vi "Begin.vi"(11 "Image Size":T1=enum."160x120") -> (0 "error out":errorcluster)   [LabVIEW 2011]
doc: "Called before other user functions, this VI is expected to open initial I/O refnums, load in file data, and do all program initialization. Notice that the <B>error out</B> terminal is simply used for data flow. Wiring it to other structures or subVIs ensures that this VI runs first."
uses:
  <vilib>/Rock Robotics/WPI/Camera/WPI_CameraImageSize.ctl
  <vilib>/Rock Robotics/SystemInterfaces/DIO/FPGA_DIOPWMChannel.ctl
  <vilib>/Rock Robotics/WPI/Joystick/WPI_JoystickDeviceEnum.ctl
  <vilib>/Rock Robotics/WPI/Camera/WPI_CameraWhite Balance Values.ctl
  <vilib>/Rock Robotics/WPI/Camera/WPI_CameraExposure Values.ctl
  <vilib>/Rock Robotics/WPI/Camera/WPI_CameraFrameRate.ctl
  <vilib>/Rock Robotics/SystemInterfaces/DIO/FPGA_DIOChannel.ctl
  <vilib>/Rock Robotics/SystemInterfaces/Typedef/FPGA_TypedefDigitalModule.ctl
  <vilib>/Rock Robotics/WPI/Encoder/WPI_EncoderType.ctl
  <vilib>/Rock Robotics/SystemInterfaces/DIO/FPGA_DIORelayChannel.ctl
  <vilib>/Rock Robotics/SystemInterfaces/Typedef/FPGA_TypedefAnalogModuleForGyro.ctl
  <vilib>/Rock Robotics/SystemInterfaces/AI/FPGA_AIGyroChannel.ctl
  <vilib>/Rock Robotics/WPI/Relay/WPI_RelayDirection.ctl
  <vilib>/Rock Robotics/WPI/MotorControl/WPI_MotorControlOpen Victor.vi
  <vilib>/Rock Robotics/WPI/RobotDrive/WPI_RobotDriveOpen4MotorWithJaguar.vi
  Robot Global Data.vi
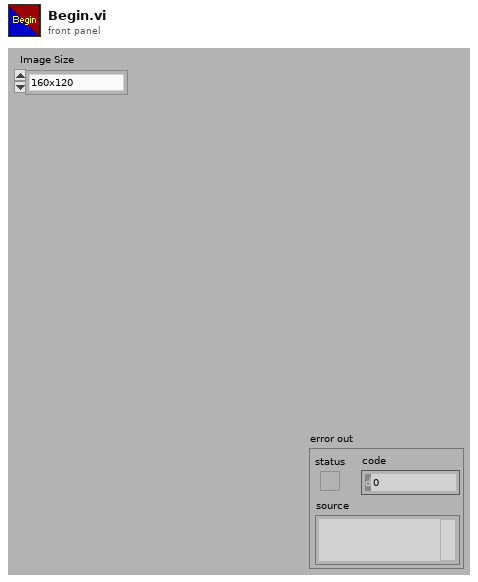
[diagram p1: front panel]
types:
  T1 = typedef "WPI_CameraImageSize.ctl" = enum16{"640x480", "320x240", "160x120"}
  T2 = typedef "WPI_RelayDirection.ctl" = enum16{"Both directions", "Forward only", "Reverse only"}
  T3 = typedef "FPGA_TypedefDigitalModule.ctl" = enum16{"Digital Module 1", "Digital Module 2"}
  T4 = typedef "FPGA_AIGyroChannel.ctl" = enum8{"AI 1", "AI 2", "Invalid"}
  T5 = typedef "FPGA_TypedefAnalogModuleForGyro.ctl" = enum16{"Analog Module 1"}
  T6 = typedef "FPGA_DIORelayChannel.ctl" = enum8{"Relay 1", "Relay 2", "Relay 3", "Relay 4", "Relay 5", "Relay 6", "Relay 7", "Relay 8", "Invalid"}
  T7 = typedef "FPGA_DIOChannel.ctl" = enum8{"DIO 1", "DIO 2", "DIO 3", "DIO 4", "DIO 5", "DIO 6", "DIO 7", "DIO 8", "DIO 9", "DIO 10", "DIO 11", "DIO 12", "DIO 13", "DIO 14", "Invalid"}
  T8 = typedef "WPI_EncoderType.ctl" = enum16{"1x", "2x", "4x"}
  T9 = typedef "FPGA_DIOPWMChannel.ctl" = enum8{"PWM 1", "PWM 2", "PWM 3", "PWM 4", "PWM 5", "PWM 6", "PWM 7", "PWM 8", "PWM 9", "PWM 10", "Invalid"}
  T10 = typedef "WPI_JoystickDeviceEnum.ctl" = enum16{"USB 1", "USB 2", "USB 3", "USB 4", "Kinect 1", "Kinect 2"}
  T11 = typedef "WPI_CameraFrameRate.ctl" = u32
  T12 = typedef "WPI_CameraExposure Values.ctl" = enum16{"Auto", "Flicker-free 50 Hz", "Flicker-free 60 Hz", "Hold current"}
  T13 = typedef "WPI_CameraWhite Balance Values.ctl" = enum16{"Auto", "Fixed indoor", "Fixed outdoor 1", "Fixed outdoor 2", "Fixed fluorescent 1", "Fixed fluorescent 2", "Hold current"}
  T14 = typedef "WPI_CameraDevRef.ctl" = cluster{"Camera Address":string, "CameraStatus":errorcluster, "Acquire Image Notifier":refnum<notifier>}
  T15 = typedef "WPI_DigitalInputDevRef.ctl" = cluster{"DevStatus":errorcluster, "DIO Channel":T7, "Digital Module":T3}
  T16 = typedef "FPGA_CounterEncoderSourceConvertionLVSourceType.ctl" = cluster{"DevStatus":errorcluster, "AnalogTriggerMode?":bool, "DigitalMode":cluster{"Digital Module":T3, "DIO Channel":T17}, "AnalogTriggerMode":cluster{"AnalogTriggerIndex":T18, "OutputType":T19}}
  T17 = typedef "FPGA_DIODigitalSourceChannel.ctl" = enum8{"DIO 1", "DIO 2", "DIO 3", "DIO 4", "DIO 5", "DIO 6", "DIO 7", "DIO 8", "DIO 9", "DIO 10", "DIO 11", "DIO 12", "DIO 13", "DIO 14", "Disabled"}
  T18 = typedef "FPGA_AnalogTriggerIndex.ctl" = enum8{"Trig 0", "Trig 1", "Trig 2", "Trig 3", "Trig 4", "Trig 5", "Trig 6", "Trig 7", "Invalid"}
  T19 = typedef "FPGA_AnalogTriggerOutType.ctl" = enum16{"InWindow", "TriggerState", "Rising", "Falling"}
  T20 = typedef "WPI_GyroDevRef.ctl" = cluster{"DevStatus":errorcluster, "Analog Module":T21, "Analog Channel":T22, "Offset":dbl, "Gain (VoltsPerDegree/Second)":dbl}
  T21 = typedef "FPGA_TypedefAnalogModule.ctl" = enum16{"Analog Module 1", "Analog Module 2"}
  T22 = typedef "FPGA_AIChannel.ctl" = enum8{"AI 1", "AI 2", "AI 3", "AI 4", "AI 5", "AI 6", "AI 7", "AI 8", "Invalid"}
  T23 = typedef "WPI_EncoderDevRef.ctl" = cluster{"DevStatus":errorcluster, "EncoderIndex":T24, "CounterIndex":T25, "DistancePerCount":dbl, "Decoding Type":T8}
  T24 = typedef "FPGA_EncoderIdx.ctl" = enum8{"Enc 0", "Enc 1", "Enc 2", "Enc 3", "Invalid"}
  T25 = typedef "FPGA_CounterCtrSystemIndex.ctl" = enum8{"Ctr 0", "Ctr 1", "Ctr 2", "Ctr 3", "Ctr 4", "Ctr 5", "Ctr 6", "Ctr 7", "Invalid"}
  T26 = typedef "WPI_RobotDriveDevRef.ctl" = cluster{"DevStatus":errorcluster, "Motors[]":T27[], "Square Inputs":bool, "Max Output":dbl, "Isochronous":bool}
  T27 = typedef "WPI_MotorControlDeviceRef.ctl" = cluster{"DeviceStatus":errorcluster, "Type":enum16{"PWM", "CAN"}, "PWM":cluster{"Digital Module":T3, "PWM Channel":T9, "DeadBand":T28}, "CAN":cluster{"Device Number":u8, "Control Mode":T29, "Semaphore":T30, "Max Vout":dbl}, "Invert":bool, "TransformRef":T31, "InvTransformRef":T31}
  T28 = typedef "WPI_PWMDeadband.ctl" = cluster{"Name":string, "maxPositivePwm":i32, "minPositivePwm":i32, "centerPwm":i32, "maxNegativePwm":i32, "minNegativePwm":i32, "angularRange":u16}
  T29 = typedef "WPI_CANJaguar_ControlMode.ctl" = enum8{"Percent VBus", "Current", "Speed", "Position", "Voltage"}
  T30 = typedef "Semaphore RefNum" = refnum<k1>
  T31 = typedef "WPI_PWMTransform_ConPane.ctl" = refnum<vi>
  T32 = typedef "WPI_RelayDevRef.ctl" = cluster{"DevStatus":errorcluster, "Relay Channel":T6, "Digital Module":T3, "Relay Direction":T2}
  T33 = typedef "WPI_JoystickDevRef.ctl" = cluster{"Device":T10}
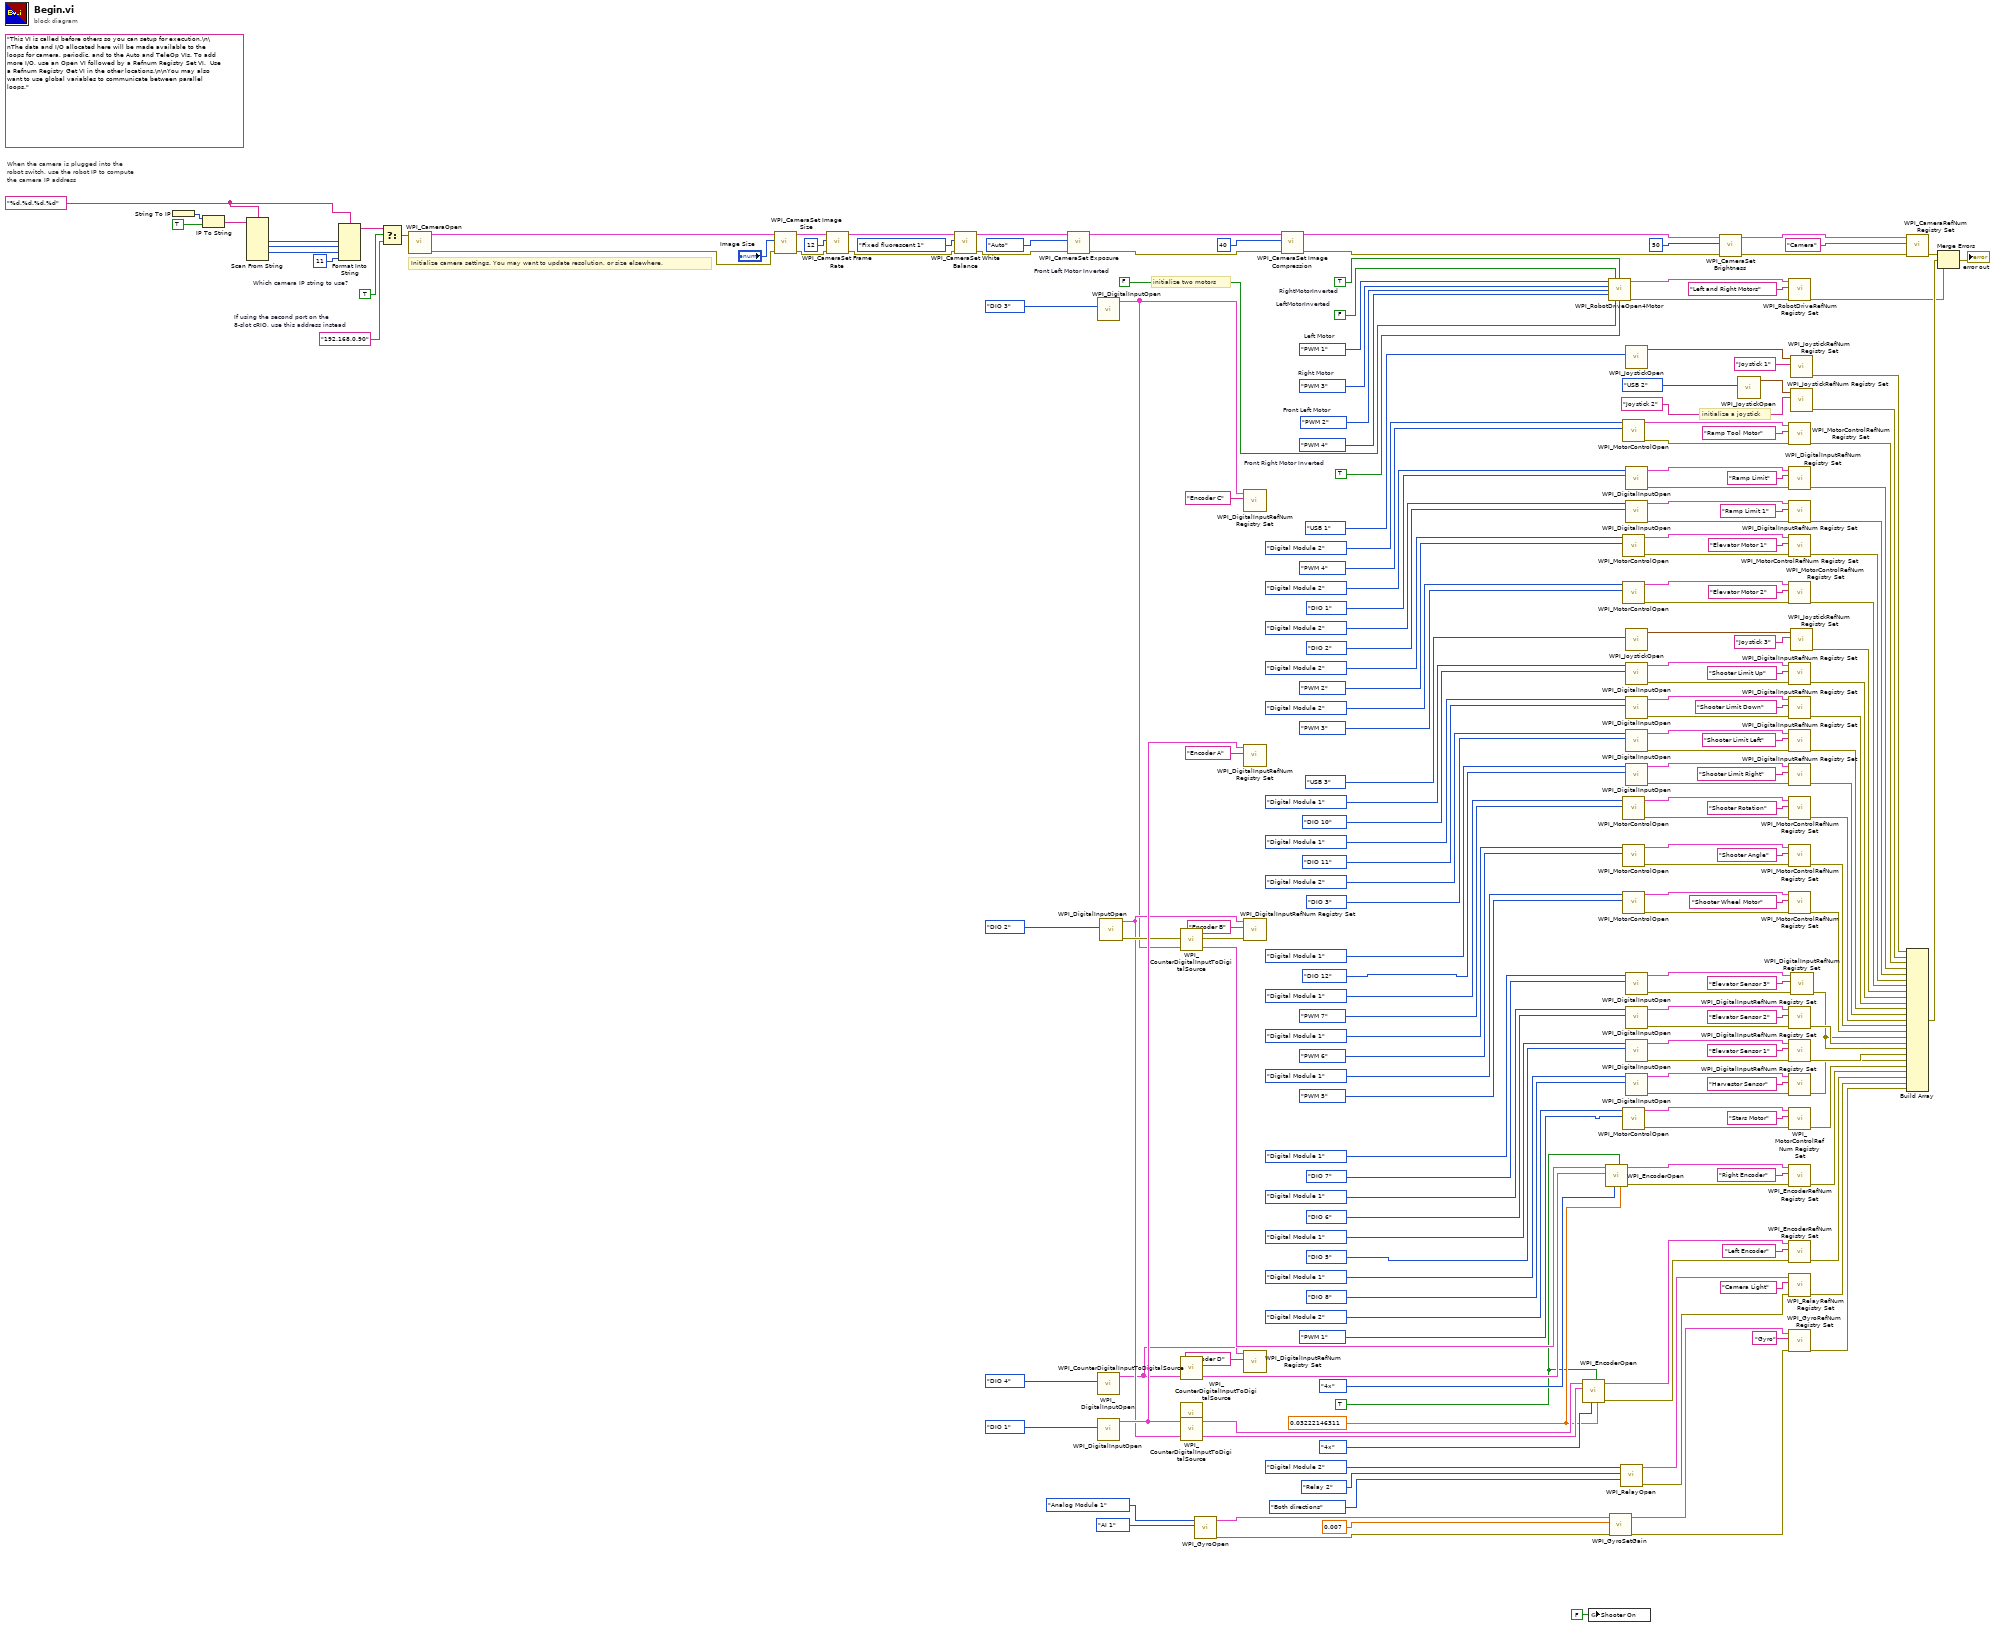
[diagram p0: block diagram]
diagram:
  w10 = FALSE  # Front Left Motor Inverted
  w11 = TRUE  # Front Right Motor Inverted
  w52 = TRUE ("External Reset Active High")
  w62 = 0.03222146311 ("DistancePerCount")
  w148 = FPGA_DIOPWMChannel."PWM 2"  # Front Left Motor
  w166 = TRUE  # Which camera IP string to use?
  w170 = "%d.%d.%d.%d" ("format string")
  (unwired) "This VI is called before others so you can setup for execution.\n\nThe data and I/O allocated here will be made available to the loops for camera, periodic, and to the Auto and TeleOp VIs. To add more I/O, use an Open VI followed by a Refnum Registry Set VI.  Use a Refnum Registry Get VI in the other locations.\n\nYou may also want to use global variables to communicate between parallel loops."
  w182 = FPGA_DIOPWMChannel."PWM 3"  # Right Motor
  w183 = FPGA_DIOPWMChannel."PWM 1"  # Left Motor
  w167 = "192.168.0.90"  # If using the second port on the 8-slot cRIO, use this address instead
  w207 = FALSE  # LeftMotorInverted
  w208 = TRUE  # RightMotorInverted
  # "When the camera is plugged into the\nrobot switch, use the robot IP to compute\nthe camera IP address"
  # "initialize a joystick"
  # "initialize two motors"
  # "Initialize camera settings. You may want to update resolution, or size elsewhere."
  n1 = String To IP() -> (0:w177:u32)  [unwired: 1 in]
  n2 = IP To String(1:TRUE ("dot notation? (F)"), 2:w177) -> (0:w175:string)
  n3 = Scan From String(format string=w170, input string=w175) -> (output 1=w174:i32, output 2=w173:i32, output 3=w172:i32)  [unwired: 7 in, 3 out]
  n4 = Format Into String(format string=w170, w174, w173, w172, 11 ("Compression")) -> (resulting string=w168:string)  [unwired: 2 in, 1 out]
  n5 = Select(t=w168, s=w166, f=w167) -> (s? t:f=w169:string)
  n6 = call <vilib>:"WPI_CameraOpen.vi"("Camera Address"=w169) -> ("error out"=w192:errorcluster, "CameraDevRef"=w193:T14)  [unwired: 1 in, 8 out]
  n7 = call <vilib>:"WPI_CameraSet Image Size.vi"("error in (no error)"=w192, "Image Size"="Image Size", "CameraDevRef"=w193) -> ("error out"=w191:errorcluster, "CameraDevRef Out"=w194:T14)  [unwired: 7 out]
  n8 = call <vilib>:"WPI_CameraSet Frame Rate.vi"("error in (no error)"=w191, "Frame Rate (fps)"=T11 12, "CameraDevRef"=w194) -> ("error out"=w190:errorcluster, "CameraDevRef Out"=w196:T14)  [unwired: 7 out]
  n9 = call <vilib>:"WPI_CameraSet White Balance.vi"("error in (no error)"=w190, "White Balance"=WPI_CameraWhite_Balance_Values."Fixed fluorescent 1", "CameraDevRef"=w196) -> ("error out"=w189:errorcluster, "CameraDevRef Out"=w195:T14)  [unwired: 7 out]
  n10 = call <vilib>:"WPI_CameraSet Exposure.vi"("error in (no error)"=w189, "Exposure"=WPI_CameraExposure_Values."Auto", "CameraDevRef"=w195) -> ("error out"=w188:errorcluster, "CameraDevRef Out"=w198:T14)  [unwired: 7 out]
  n11 = call <vilib>:"WPI_DigitalInputOpen.vi"("DIO Channel"=FPGA_DIOChannel."DIO 3") -> ("DigitalInputDevRef"=w56:T15)  [unwired: 2 in, 8 out]
  n12 = call <vilib>:"WPI_DigitalInputOpen.vi"("DIO Channel"=FPGA_DIOChannel."DIO 4") -> ("DigitalInputDevRef"=w55:T15)  [unwired: 2 in, 8 out]
  n13 = call <vilib>:"WPI_DigitalInputOpen.vi"("DIO Channel"=FPGA_DIOChannel."DIO 1") -> ("DigitalInputDevRef"=w61:T15)  [unwired: 2 in, 8 out]
  n14 = call <vilib>:"WPI_DigitalInputOpen.vi"("DIO Channel"=FPGA_DIOChannel."DIO 2") -> ("error out"=w59:errorcluster, "DigitalInputDevRef"=w58:T15)  [unwired: 2 in, 7 out]
  n15 = call <vilib>:"WPI_CounterDigitalInputToDigitalSource.vi"("DigitalInputDevRef"=w56) -> ("Digital Source"=w65:T16)  [unwired: 6 out]
  n16 = call <vilib>:"WPI_CounterDigitalInputToDigitalSource.vi"("DigitalInputDevRef"=w55) -> ("Digital Source"=w63:T16)  [unwired: 6 out]
  n17 = call <vilib>:"WPI_CounterDigitalInputToDigitalSource.vi"("DigitalInputDevRef"=w61) -> ("Digital Source"=w69:T16)  [unwired: 6 out]
  n18 = call <vilib>:"WPI_CounterDigitalInputToDigitalSource.vi"("DigitalInputDevRef"=w58) -> ("Digital Source"=w68:T16)  [unwired: 6 out]
  n19 = call <vilib>:"WPI_GyroOpen.vi"("Analog Channel"=FPGA_AIGyroChannel."AI 1", "Analog Module (Module 1)"=FPGA_TypedefAnalogModuleForGyro."Analog Module 1" ("Analog Module (Slot 1)")) -> ("error out"=w16:errorcluster, "GyroDevRef"=w20:T20)  [unwired: 4 in, 4 out]
  n20 = call <vilib>:"WPI_DigitalInputRefNum Registry Set.vi"("refnum name"="Encoder C", "DigitalInputDevRef"=w56) -> ()  [unwired: 1 in, 9 out]
  n21 = call <vilib>:"WPI_DigitalInputRefNum Registry Set.vi"("refnum name"="Encoder A", "DigitalInputDevRef"=w61) -> ()  [unwired: 1 in, 9 out]
  n22 = call <vilib>:"WPI_DigitalInputRefNum Registry Set.vi"("error in (no error)"=w59, "refnum name"="Encoder B", "DigitalInputDevRef"=w58) -> ()  [unwired: 9 out]
  n23 = call <vilib>:"WPI_DigitalInputRefNum Registry Set.vi"("refnum name"="Encoder D", "DigitalInputDevRef"=w55) -> ()  [unwired: 1 in, 9 out]
  n24 = call <vilib>:"WPI_CameraSet Image Compression.vi"("error in (no error)"=w188, "Compression"=40, "CameraDevRef"=w198) -> ("error out"=w187:errorcluster, "CameraDevRef Out"=w197:T14)  [unwired: 7 out]
  n25 = call <vilib>:"WPI_EncoderOpen.vi"("DistancePerCount"=w62, "External Reset Active High"=w52, "Decoding Type"=WPI_EncoderType."4x", "BSource"=w68, "ASource"=w69) -> ("error out"=w77:errorcluster, "EncoderDevRef"=w76:T23)  [unwired: 3 in, 2 out]
  n26 = global write "Robot Global Data.vi" "Shooter On"(FALSE ("Shooter On")) -> ()
  n27 = call <vilib>:"WPI_EncoderOpen.vi"("DistancePerCount"=w62, "External Reset Active High"=w52, "Decoding Type"=WPI_EncoderType."4x", "BSource"=w63, "ASource"=w65) -> ("error out"=w75:errorcluster, "EncoderDevRef"=w74:T23)  [unwired: 3 in, 2 out]
  n28 = call-poly <vilib>:"WPI_RobotDriveOpen4Motor.vi"("Rear Left Motor"=w183, "Rear Left Motor Inverted"=w207, "Rear Right Motor Inverted"=w208, "Rear Right Motor"=w182, "Front Left Motor"=w148, "Front Right Motor"=FPGA_DIOPWMChannel."PWM 4", "Front Left Motor Inverted"=w10, "Front Right Motor Inverted"=w11) -> ("RobotDriveDevRef"=w205:T26, "error out"=w201:errorcluster)  [unwired: 6 in]
  n29 = call <vilib>:"WPI_GyroSetGain.vi"("error in (no error)"=w16, "Gain (VoltsPerDegree/Second)"=0.007, "GyroDevRef"=w20) -> ("error out"=w15:errorcluster, "GyroDevRef"=w17:T20)  [unwired: 7 out]
  n30 = call <vilib>:"WPI_RelayOpen.vi"("Relay Direction"=WPI_RelayDirection."Both directions", "Relay Channel"=FPGA_DIORelayChannel."Relay 2", "Digital Module (Module 1)"=FPGA_TypedefDigitalModule."Digital Module 2") -> ("error out"=w24:errorcluster, "RelayDevRef"=w25:T32)  [unwired: 7 in]
  n31 = call-poly <vilib>:"WPI_MotorControlOpen.vi"("PWM Channel"=FPGA_DIOPWMChannel."PWM 4", "Digital Module (Module 1)"=FPGA_TypedefDigitalModule."Digital Module 2") -> ("error out"=w161:errorcluster, "MotorControlDeviceRef"=w162:T27)  [unwired: 8 in]
  n32 = call-poly <vilib>:"WPI_MotorControlOpen.vi"("PWM Channel"=FPGA_DIOPWMChannel."PWM 2", "Digital Module (Module 1)"=FPGA_TypedefDigitalModule."Digital Module 2") -> ("error out"=w144:errorcluster, "MotorControlDeviceRef"=w146:T27)  [unwired: 8 in]
  n33 = call-poly <vilib>:"WPI_MotorControlOpen.vi"("PWM Channel"=FPGA_DIOPWMChannel."PWM 3", "Digital Module (Module 1)"=FPGA_TypedefDigitalModule."Digital Module 2") -> ("error out"=w141:errorcluster, "MotorControlDeviceRef"=w143:T27)  [unwired: 8 in]
  n34 = call-poly <vilib>:"WPI_MotorControlOpen.vi"("PWM Channel"=FPGA_DIOPWMChannel."PWM 7", "Digital Module (Module 1)"=FPGA_TypedefDigitalModule."Digital Module 1") -> ("error out"=w117:errorcluster, "MotorControlDeviceRef"=w118:T27)  [unwired: 8 in]
  n35 = call-poly <vilib>:"WPI_MotorControlOpen.vi"("PWM Channel"=FPGA_DIOPWMChannel."PWM 6", "Digital Module (Module 1)"=FPGA_TypedefDigitalModule."Digital Module 1") -> ("error out"=w112:errorcluster, "MotorControlDeviceRef"=w113:T27)  [unwired: 8 in]
  n36 = call-poly <vilib>:"WPI_MotorControlOpen.vi"("PWM Channel"=FPGA_DIOPWMChannel."PWM 5", "Digital Module (Module 1)"=FPGA_TypedefDigitalModule."Digital Module 1") -> ("error out"=w108:errorcluster, "MotorControlDeviceRef"=w109:T27)  [unwired: 8 in]
  n37 = call-poly <vilib>:"WPI_MotorControlOpen.vi"("PWM Channel"=FPGA_DIOPWMChannel."PWM 1", "Digital Module (Module 1)"=FPGA_TypedefDigitalModule."Digital Module 2") -> ("error out"=w80:errorcluster, "MotorControlDeviceRef"=w81:T27)  [unwired: 8 in]
  n38 = call <vilib>:"WPI_JoystickOpen.vi"("JoystickDevice"=WPI_JoystickDeviceEnum."USB 1") -> ("JoystickDevRef"=w203:T33)  [unwired: 10 out]
  n39 = call <vilib>:"WPI_DigitalInputOpen.vi"("DIO Channel"=FPGA_DIOChannel."DIO 1", "Digital Module (Module 1)"=FPGA_TypedefDigitalModule."Digital Module 2") -> ("error out"=w157:errorcluster, "DigitalInputDevRef"=w156:T15)  [unwired: 8 in]
  n40 = call <vilib>:"WPI_DigitalInputOpen.vi"("DIO Channel"=FPGA_DIOChannel."DIO 2", "Digital Module (Module 1)"=FPGA_TypedefDigitalModule."Digital Module 2") -> ("error out"=w153:errorcluster, "DigitalInputDevRef"=w152:T15)  [unwired: 8 in]
  n41 = call <vilib>:"WPI_JoystickOpen.vi"("JoystickDevice"=WPI_JoystickDeviceEnum."USB 3") -> ("JoystickDevRef"=w136:T33)  [unwired: 10 out]
  n42 = call <vilib>:"WPI_DigitalInputOpen.vi"("DIO Channel"=FPGA_DIOChannel."DIO 10", "Digital Module (Module 1)"=FPGA_TypedefDigitalModule."Digital Module 1") -> ("error out"=w100:errorcluster, "DigitalInputDevRef"=w133:T15)  [unwired: 8 in]
  n43 = call <vilib>:"WPI_DigitalInputOpen.vi"("DIO Channel"=FPGA_DIOChannel."DIO 11", "Digital Module (Module 1)"=FPGA_TypedefDigitalModule."Digital Module 1") -> ("error out"=w99:errorcluster, "DigitalInputDevRef"=w129:T15)  [unwired: 8 in]
  n44 = call <vilib>:"WPI_DigitalInputOpen.vi"("DIO Channel"=FPGA_DIOChannel."DIO 3", "Digital Module (Module 1)"=FPGA_TypedefDigitalModule."Digital Module 2") -> ("error out"=w98:errorcluster, "DigitalInputDevRef"=w125:T15)  [unwired: 8 in]
  n45 = call <vilib>:"WPI_DigitalInputOpen.vi"("DIO Channel"=FPGA_DIOChannel."DIO 12", "Digital Module (Module 1)"=FPGA_TypedefDigitalModule."Digital Module 1") -> ("error out"=w97:errorcluster, "DigitalInputDevRef"=w121:T15)  [unwired: 8 in]
  n46 = call <vilib>:"WPI_DigitalInputOpen.vi"("DIO Channel"=FPGA_DIOChannel."DIO 7", "Digital Module (Module 1)"=FPGA_TypedefDigitalModule."Digital Module 1") -> ("error out"=w96:errorcluster, "DigitalInputDevRef"=w104:T15)  [unwired: 8 in]
  n47 = call <vilib>:"WPI_DigitalInputOpen.vi"("DIO Channel"=FPGA_DIOChannel."DIO 6", "Digital Module (Module 1)"=FPGA_TypedefDigitalModule."Digital Module 1") -> ("error out"=w91:errorcluster, "DigitalInputDevRef"=w95:T15)  [unwired: 8 in]
  n48 = call <vilib>:"WPI_DigitalInputOpen.vi"("DIO Channel"=FPGA_DIOChannel."DIO 5", "Digital Module (Module 1)"=FPGA_TypedefDigitalModule."Digital Module 1") -> ("error out"=w87:errorcluster, "DigitalInputDevRef"=w90:T15)  [unwired: 8 in]
  n49 = call <vilib>:"WPI_DigitalInputOpen.vi"("DIO Channel"=FPGA_DIOChannel."DIO 8", "Digital Module (Module 1)"=FPGA_TypedefDigitalModule."Digital Module 1") -> ("error out"=w82:errorcluster, "DigitalInputDevRef"=w86:T15)  [unwired: 8 in]
  n50 = call <vilib>:"WPI_CameraSet Brightness.vi"("error in (no error)"=w187, "Brightness"=50, "CameraDevRef"=w197) -> ("error out"=w185:errorcluster, "CameraDevRef Out"=w186:T14)  [unwired: 7 out]
  n51 = call <vilib>:"WPI_JoystickOpen.vi"("JoystickDevice"=WPI_JoystickDeviceEnum."USB 2") -> ("JoystickDevRef"=w165:T33)  [unwired: 10 in]
  n52 = call <vilib>:"WPI_RobotDriveRefNum Registry Set.vi"("error in (no error)"=w201, "refnum name"="Left and Right Motors", "RobotDriveDevRef"=w205) -> ("error out"=w2:errorcluster)  [unwired: 8 out]
  n53 = call <vilib>:"WPI_MotorControlRefNum Registry Set.vi"("error in (no error)"=w161, "refnum name"="Ramp Tool Motor", "MotorControlDevRef"=w162) -> ("error out"=w48:errorcluster)  [unwired: 7 in, 1 out]
  n54 = call <vilib>:"WPI_DigitalInputRefNum Registry Set.vi"("error in (no error)"=w157, "refnum name"="Ramp Limit", "DigitalInputDevRef"=w156) -> ("error out"=w47:errorcluster)  [unwired: 7 in, 1 out]
  n55 = call <vilib>:"WPI_DigitalInputRefNum Registry Set.vi"("error in (no error)"=w153, "refnum name"="Ramp Limit 1", "DigitalInputDevRef"=w152) -> ("error out"=w46:errorcluster)  [unwired: 7 in, 1 out]
  n56 = call <vilib>:"WPI_MotorControlRefNum Registry Set.vi"("error in (no error)"=w144, "refnum name"="Elevator Motor 1", "MotorControlDevRef"=w146) -> ("error out"=w45:errorcluster)  [unwired: 7 in, 1 out]
  n57 = call <vilib>:"WPI_MotorControlRefNum Registry Set.vi"("error in (no error)"=w141, "refnum name"="Elevator Motor 2", "MotorControlDevRef"=w143) -> ("error out"=w44:errorcluster)  [unwired: 7 in, 1 out]
  n58 = call <vilib>:"WPI_DigitalInputRefNum Registry Set.vi"("error in (no error)"=w100, "refnum name"="Shooter Limit Up", "DigitalInputDevRef"=w133) -> ("error out"=w42:errorcluster)  [unwired: 7 in, 1 out]
  n59 = call <vilib>:"WPI_DigitalInputRefNum Registry Set.vi"("error in (no error)"=w99, "refnum name"="Shooter Limit Down", "DigitalInputDevRef"=w129) -> ("error out"=w41:errorcluster)  [unwired: 7 in, 1 out]
  n60 = call <vilib>:"WPI_DigitalInputRefNum Registry Set.vi"("error in (no error)"=w98, "refnum name"="Shooter Limit Left", "DigitalInputDevRef"=w125) -> ("error out"=w40:errorcluster)  [unwired: 7 in, 1 out]
  n61 = call <vilib>:"WPI_DigitalInputRefNum Registry Set.vi"("error in (no error)"=w97, "refnum name"="Shooter Limit Right", "DigitalInputDevRef"=w121) -> ("error out"=w39:errorcluster)  [unwired: 7 in, 1 out]
  n62 = call <vilib>:"WPI_MotorControlRefNum Registry Set.vi"("error in (no error)"=w117, "refnum name"="Shooter Rotation", "MotorControlDevRef"=w118) -> ("error out"=w38:errorcluster)  [unwired: 7 in, 1 out]
  n63 = call <vilib>:"WPI_MotorControlRefNum Registry Set.vi"("error in (no error)"=w112, "refnum name"="Shooter Angle", "MotorControlDevRef"=w113) -> ("error out"=w37:errorcluster)  [unwired: 7 in, 1 out]
  n64 = call <vilib>:"WPI_MotorControlRefNum Registry Set.vi"("error in (no error)"=w108, "refnum name"="Shooter Wheel Motor", "MotorControlDevRef"=w109) -> ("error out"=w36:errorcluster)  [unwired: 7 in, 1 out]
  n65 = call <vilib>:"WPI_DigitalInputRefNum Registry Set.vi"("error in (no error)"=w91, "refnum name"="Elevator Sensor 2", "DigitalInputDevRef"=w95) -> ("error out"=w35:errorcluster)  [unwired: 7 in, 1 out]
  n66 = call <vilib>:"WPI_DigitalInputRefNum Registry Set.vi"("error in (no error)"=w87, "refnum name"="Elevator Sensor 1", "DigitalInputDevRef"=w90) -> ("error out"=w33:errorcluster)  [unwired: 7 in, 1 out]
  n67 = call <vilib>:"WPI_DigitalInputRefNum Registry Set.vi"("error in (no error)"=w82, "refnum name"="Harvestor Sensor", "DigitalInputDevRef"=w86) -> ("error out"=w32:errorcluster)  [unwired: 7 in, 1 out]
  n68 = call <vilib>:"WPI_MotorControlRefNum Registry Set.vi"("error in (no error)"=w80, "refnum name"="Stars Motor", "MotorControlDevRef"=w81) -> ("error out"=w31:errorcluster)  [unwired: 7 in, 1 out]
  n69 = call <vilib>:"WPI_EncoderRefNum Registry Set.vi"("error in (no error)"=w75, "refnum name"="Right Encoder", "EncoderDevRef"=w74) -> ("error out"=w30:errorcluster)  [unwired: 8 out]
  n70 = call <vilib>:"WPI_EncoderRefNum Registry Set.vi"("error in (no error)"=w77, "refnum name"="Left Encoder", "EncoderDevRef"=w76) -> ("error out"=w29:errorcluster)  [unwired: 8 out]
  n71 = call <vilib>:"WPI_RelayRefNum Registry Set.vi"("error in (no error)"=w24, "refnum name"="Camera Light", "RelayDevRef"=w25) -> ("error out"=w21:errorcluster)  [unwired: 7 in, 1 out]
  n72 = call <vilib>:"WPI_GyroRefNum Registry Set.vi"("error in (no error)"=w15, "refnum name"="Gyro", "GyroDevRef"=w17) -> ("error out"=w12:errorcluster)  [unwired: 8 out]
  n73 = call <vilib>:"WPI_JoystickRefNum Registry Set.vi"("refnum name"="Joystick 1", "JoystickDevRef"=w203) -> ("error out"=w50:errorcluster)  [unwired: 1 in, 8 out]
  n74 = call <vilib>:"WPI_JoystickRefNum Registry Set.vi"("refnum name"="Joystick 2", "JoystickDevRef"=w165) -> ("error out"=w49:errorcluster)  [unwired: 8 in, 1 out]
  n75 = call <vilib>:"WPI_JoystickRefNum Registry Set.vi"("refnum name"="Joystick 3", "JoystickDevRef"=w136) -> ("error out"=w43:errorcluster)  [unwired: 1 in, 8 out]
  n76 = call <vilib>:"WPI_DigitalInputRefNum Registry Set.vi"("error in (no error)"=w96, "refnum name"="Elevator Sensor 3", "DigitalInputDevRef"=w104) -> ("error out"=w34:errorcluster)  [unwired: 7 in, 1 out]
  n77 = call <vilib>:"WPI_CameraRefNum Registry Set.vi"("error in (no error)"=w185, "refnum name"="Camera", "CameraDevRef"=w186) -> ("error out"=w26:errorcluster)  [unwired: 8 out]
  n78 = Build Array(w50, w49, w48, w47, w46, w45, w44, w43, w42, w41, w40, w39, w38, w37, w36, w34, w35, w34, w33, w32, w31, w30, w29, w21, w12) -> (w27:errorcluster[])
  n79 = Merge Errors(w26, w27, w2) -> (→"error out":errorcluster)
